vi "S2C_VLFT10_Proc_ExtractTargz.vi"(8 "Error In":errorcluster, 11 "Paths":string) -> (0 "Error Out":errorcluster, 3 "Result":string)   [LabVIEW 2015]
uses:
  <vilib>/regexp/Match Regular Expression.xnode
panel:
  in  "PassMatch":string="Everything is Ok[\\s\\S]*?Everything is Ok"
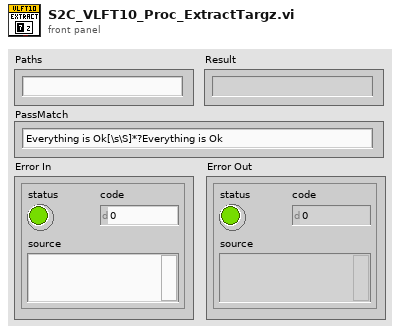
[diagram p1: front panel]
types:
  T1 = cluster{"7zip Path":string, "Targz Path":string, "Temp Path":string}
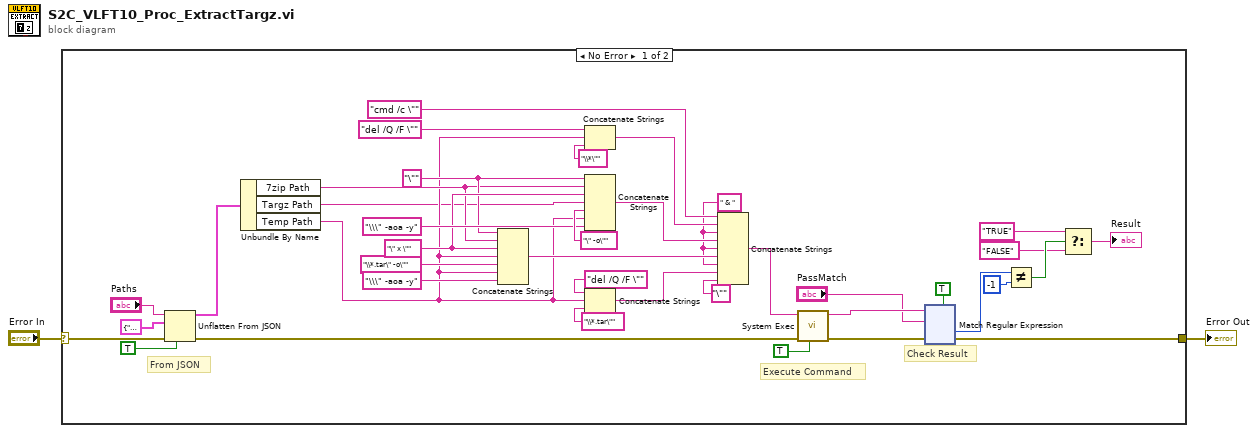
[diagram p0: block diagram]
diagram:
  n1 = case shown="No Error" "Error In" {
    selector: "Error In" -> [w41 w156]
    tunnel: [w17 w156] -> w1
    frame No Error {
      w30 = "\"" ("string")
      w24 = " & " ("string")
      w35 = "\" x \"" ("string")
      # "From JSON"
      # "Check Result"
      # "Execute Command"
      n2 = Unflatten From JSON(JSON string="Paths", type and defaults=T1 {"7zip Path"="", "Targz Path"="", "Temp Path"=""}, default null elements? (F)=TRUE, error in (no error)=w41) -> (value=w11:T1, error out=w23:errorcluster)  [unwired: 3 in]
      n3 = Unbundle By Name(w11) -> ("7zip Path"=w10:string, "Targz Path"=w8:string, "Temp Path"=w9:string)
      n4 = Concatenate Strings(w30, w10, w35, w9, "\\*.tar\" -o\"" ("string"), w9, "\\\" -aoa -y" ("string")) -> (w31:string)
      n5 = Concatenate Strings("del /Q /F \"" ("string"), w9, "\\*\"" ("string")) -> (w37:string)
      n6 = Concatenate Strings(w30, w10, w35, w8, "\" -o\"" ("string"), w9, "\\\" -aoa -y" ("string")) -> (w32:string)
      n7 = Concatenate Strings("del /Q /F \"" ("string"), w9, "\\*.tar\"" ("string")) -> (w25:string)
      n8 = Concatenate Strings("cmd /c \"" ("string"), w37, w24, w32, w24, w31, w24, w25, "\"" ("string")) -> (w21:string)
      n9 = call <vilib>:"System Exec.vi"("run minimized? (F)"=TRUE, "error in (no error)"=w23, "command line"=w21) -> ("error out"=w20:errorcluster, "standard output"=w15:string)  [unwired: 5 in, 2 out]
      n10 = xnode "Match Regular Expression"("input string"=w15, "regular expression"="PassMatch", "error in"=w20, "multiline? (F)"=TRUE) -> ("offset past match"=w16:i32, "error out"=w17:errorcluster)  [unwired: 2 in, 3 out]
      n11 = Not Equal?(x=w16, y=-1) -> (x != y?=w14:bool)
      n12 = Select(t="TRUE", s=w14, f="FALSE") -> (s? t:f=→"Result":string)
    }
    frame Error {
    }
  }
  "Error Out" <- w1
